vi "Set Analog Edge Trigger.vi"(7 "Trigger Direction":T2, 8 "error in (no error)":errorcluster, 10 "Analog Trigger":T1, 11 "Item Ref in":T3 format="%.0x") -> (0 "error out":errorcluster, 3 "Item Ref out":T3 format="%.0x")   [LabVIEW 2012, in "Waveform Data Logger Shared.lvlib"]
uses:
  Waveform Data Logger Shared.lvlib
  <vilib>/NI Veristand/Custom Device API/Custom Device Item Ref.ctl
  Types/Trigger Direction.ctl
  Types/Analog Trigger.ctl
  Globals/Property Strings.vi
  <vilib>/NI Veristand/Custom Device API/Set Item Property (Boolean).vi
  <vilib>/NI Veristand/Custom Device API/Set Item Property (U16).vi
  <vilib>/NI Veristand/Custom Device API/Set Item Property (Double).vi
  <vilib>/NI VeriStand/Custom Device API/Custom Device API.lvlib
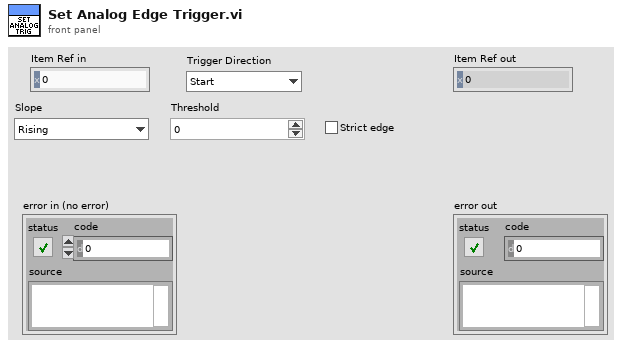
[diagram p1: front panel]
types:
  T1 = typedef "Waveform Data Logger Shared.lvlib/Analog Trigger.ctl" = cluster{"Strict edge":bool, "Slope":enum16{"Rising", "Falling"}, "Threshold":dbl}
  T2 = typedef "Waveform Data Logger Shared.lvlib/Trigger Direction.ctl" = enum16{"Start", "Stop"}
  T3 = typedef "Custom Device API.lvlib/Custom Device Item Ref.ctl" = u64
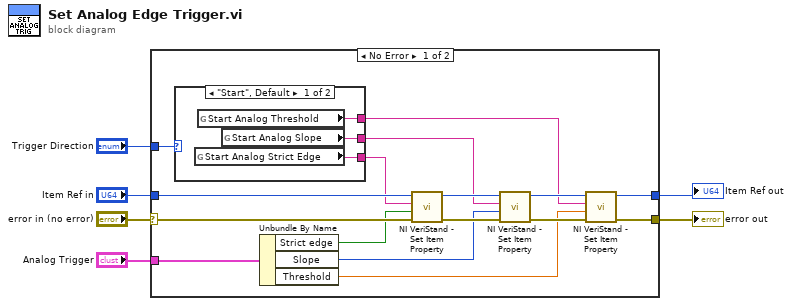
[diagram p0: block diagram]
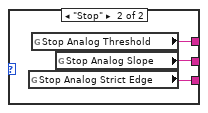
[diagram p2: hidden frame]
diagram:
  n1 = case shown="No Error" "error in (no error)" {
    selector: "error in (no error)" -> [w18 w29]
    tunnel: [w10 w30] -> w6
    tunnel: [w9 w29] -> w5
    tunnel: "Item Ref in" -> [w20 w30]
    tunnel: "Analog Trigger" -> [w19 _]
    tunnel: "Trigger Direction" -> [w17 _]
    frame No Error {
      n2 = case shown="\"Start\", Default" w17 {
        tunnel: [w25 w27] -> w13
        tunnel: [w24 w26] -> w14
        tunnel: [w23 w28] -> w7
        frame "Start", Default {
          n3 = global read "Property Strings.vi" "Start Analog Strict Edge"() -> (w24:string)
          n4 = global read "Property Strings.vi" "Start Analog Threshold"() -> (w23:string)
          n5 = global read "Property Strings.vi" "Start Analog Slope"() -> (w25:string)
        }
        frame "Stop" {
          n6 = global read "Property Strings.vi" "Stop Analog Strict Edge"() -> (w26:string)
          n7 = global read "Property Strings.vi" "Stop Analog Threshold"() -> (w28:string)
          n8 = global read "Property Strings.vi" "Stop Analog Slope"() -> (w27:string)
        }
      }
      n9 = Unbundle By Name(w19) -> ("Strict edge"=w16:bool, "Slope"=w15:enum16{"Rising", "Falling"}, "Threshold"=w8:dbl)
      n10 = call-poly <vilib>:"NI VeriStand - Set Item Property.vi"("error in (no error)"=w18, "Value"=w16, "Property Name"=w14, "Item Ref in"=w20) -> ("error out"=w22:errorcluster, "Item Ref out"=w21:T3)  [unwired: 5 in, 1 out]
      n11 = call-poly <vilib>:"NI VeriStand - Set Item Property.vi"("error in (no error)"=w22, "Value"=w15, "Property Name"=w13, "Item Ref in"=w21) -> ("error out"=w11:errorcluster, "Item Ref out"=w12:T3)  [unwired: 5 in, 1 out]
      n12 = call-poly <vilib>:"NI VeriStand - Set Item Property.vi"("error in (no error)"=w11, "Value"=w8, "Property Name"=w7, "Item Ref in"=w12) -> ("error out"=w9:errorcluster, "Item Ref out"=w10:T3)  [unwired: 5 in, 1 out]
    }
    frame Error {
    }
  }
  "Item Ref out" <- w6
  "error out" <- w5
